vi "startTime.get.vi"(8 "error in (no error)":errorcluster, 11 "Run in":refnum<class "Run.lvclass">) -> (0 "error out":errorcluster, 2 "startTime":timestamp format="%<%x %.3X>T", 3 "Run out":refnum<class "Run.lvclass">)   [LabVIEW 2020, in "Run.lvclass"]
uses:
  Run.lvclass
  Run.lvclass/Run.ctl
  20fa2b38-31a7-4466-a6b6-6ae4e02b8116.vi
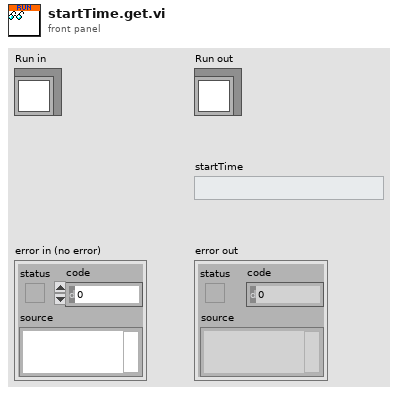
[diagram p1: front panel]
types:
  T1 = cluster{"secondsSinceEpoch":i32, "offsetNanoseconds":i32}
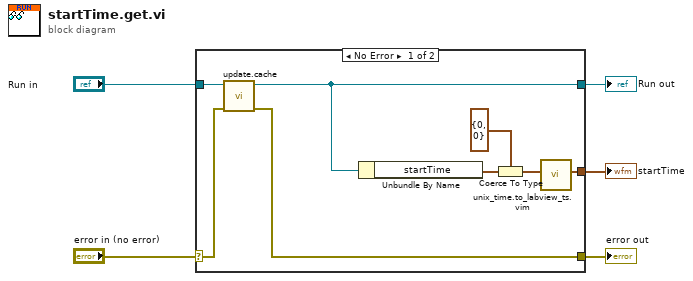
[diagram p0: block diagram]
diagram:
  n1 = case shown="No Error" "error in (no error)" {
    selector: "error in (no error)" -> [w13 w14]
    tunnel: [w8 w14] -> w4
    tunnel: [w6 w15] -> w2
    tunnel: "Run in" -> [w7 w15]
    tunnel: [w12 _] -> w1
    frame No Error {
      n2 = call "update.cache.vi"("error in"=w13, "Run in"=w7) -> ("error out"=w8:errorcluster, "Run out"=w6:refnum<class "Run.lvclass">)  [unwired: 8 in]
      n3 = Unbundle By Name(w6) -> ("startTime"=w10:T1)
      n4 = Coerce To Type(0:w10, 1:cluster{"Seconds":i32, "Nanoseconds":i32} {"Seconds"=0, "Nanoseconds"=0} ("UNIX Timestamp")) -> (2:w9:cluster{"Seconds":i32, "Nanoseconds":i32})
      n5 = call "unix_time.to_labview_ts.vim"("UNIX Timestamp"=w9) -> ("Time Stamp"=w12:timestamp)  [unwired: 10 in]
    }
    frame Error {
    }
  }
  "error out" <- w4
  "Run out" <- w2
  "startTime" <- w1
